vi "AddUserToDB.vi"(6 "DatabaseConnectionInfo":T1, 7 "Name":string, 8 "error in (no error)":errorcluster, 9 "Password":string, 10 "Username":string, 11 "Surname":string) -> (0 "error out":errorcluster)   [LabVIEW 2017]
uses:
  <vilib>/addons/database/Connection.llb/DB Tools Open Connec (Path).vi
  <vilib>/addons/database/NI_Database_API.lvlib
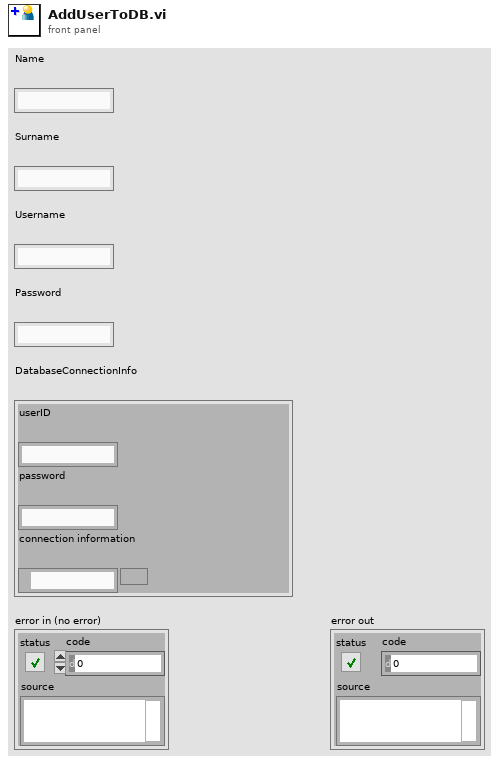
[diagram p1: front panel]
types:
  T1 = cluster{"userID":string, "password":string, "connection information":path}
  T2 = cluster{"Name":string, "Surname":string, "Username":string, "Password":string}
  T3 = typedef "NI_Database_API.lvlib/Conn ObjectReference.ctl" = refnum<k1>
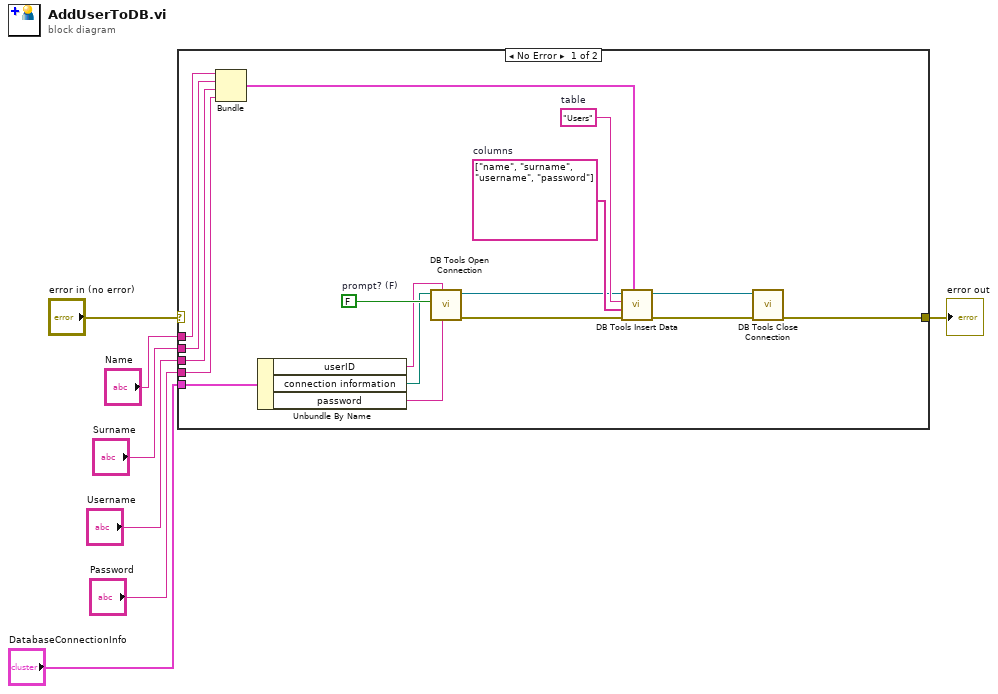
[diagram p0: block diagram]
diagram:
  n1 = case shown="No Error" "error in (no error)" {
    selector: "error in (no error)" -> [_ w25]
    tunnel: [w24 w25] -> w6
    tunnel: "DatabaseConnectionInfo" -> [w23 _]
    tunnel: "Name" -> [w11 _]
    tunnel: "Surname" -> [w10 _]
    tunnel: "Username" -> [w9 _]
    tunnel: "Password" -> [w8 _]
    frame No Error {
      w17 = string[] ["name", "surname", "username", "password"]  # columns
      w18 = "Users"  # table
      w22 = FALSE  # prompt? (F)
      n2 = Bundle("Name"=w11, "Surname"=w10, "Username"=w9, "Password"=w8) -> (w12:T2)  [unwired: 1 in]
      n3 = Unbundle By Name(w23) -> ("userID"=w21:string, "connection information"=w19:path, "password"=w20:string)
      n4 = call-poly <vilib>:"DB Tools Open Connection.vi"("password"=w20, "userID"=w21, "prompt? (F)"=w22, "connection information"=w19) -> ("error out"=w15:errorcluster, "connection reference"=w16:T3)  [unwired: 4 in]
      n5 = call <vilib>:"DB Tools Insert Data.vi"("data"=w12, "error in (no error)"=w15, "columns"=w17, "table"=w18, "connection reference"=w16) -> ("error out"=w14:errorcluster, "connection reference out"=w13:T3)  [unwired: 5 in]
      n6 = call <vilib>:"DB Tools Close Connection.vi"("error in (no error)"=w14, "connection reference"=w13) -> ("error out"=w24:errorcluster)  [unwired: 5 in]
    }
    frame Error {
    }
  }
  "error out" <- w6
